vi "OAT Track Orders in Resampled Signal (Single Channel).vi"(0 "resampled signal":cluster{"r0":dbl, "dr":dbl, "Y":dbl[]}={"r0"=0.0, "dr"=1.0, "Y"=[]} {"r0" format="%.2p"; "dr" format="%.2p"; "Y" format="%.2f"}, 1 "orders (1.0)":dbl[](array[numeric])=[1.0] format="%.2f", 2 "X axis selection":u16(ring)=2 items=["Time", "Revolution", "RPM"], 3 "reset? (True)":bool=TRUE, 5 "channel info":T1={"sensor sensitivity"=1000.0, "engineering units"=1, "dB reference"=1.0, "custom label"="EU", "weighting filter"=0, "pregain"=0.0} {"pregain" format="%.2f"; "weighting filter" items=["Linear", "A-weighting", "B-weighting", "C-weighting", "ITU-R 468-4", "Dolby", "CCITT", "C-message", "Wb", "Wc", "Wd", "We", "Wf", "Wh", "Wj", "Wk", "Wm", "AES17 20 kHz lowpass", "AES17 40 kHz lowpass", "AES17 20 kHz highpass", "AES17 40 kHz highpass"]; "dB reference" format="%^.1e"; "engineering units" items=["custom..."=0, "V"=1, "A"=21, "C"=30, "pC"=31, "s"=32, "-"=29, "Pa"=2, "N"=20, "g"=3, "m/s^2"=4, "m/s"=5, "m"=6, "mm/s"=12, "mm"=13, "micron/s"=14, "micron"=15, "in/s^2"=7, "in/s"=8, "in"=9, "mil/s"=10, "mil"=11, "rad/s^2"=16, "rad/s"=17, "rad"=18, "deg/s^2"=26, "deg/s"=27, "deg"=28, "RPM"=22, "cycle/s^2"=23, "Hz"=24, "cycle"=25, "strain"=19]; "sensor sensitivity" format="%#_5f"}, 7 "time instant":dbl[](array[numeric]) format="%.2f", 11 "error in (no error)":errorcluster, 12 "bandwidth [order]":dbl format="%.2f", 13 "phase setting":T5) -> (4 "magnitudes (RMS)":cluster{"X":dbl[], "Y":dbl[]}[](array[cluster]) {"Y" format="%.2f"; "X" format="%.2f"}, 6 "phase lags":cluster{"X":dbl[], "Y":dbl[]}[](array[cluster]) {"Y" format="%.2f"; "X" format="%.2f"}, 8 "samples/rev":dbl format="%.2f", 10 "unit labels":T4, 15 "error out":errorcluster)   [LabVIEW 2017]
doc: "Computes magnitudes and phases for designated orders from <B>resampled signal</B>."
uses:
  <vilib>/addons/_NISVFA/_Shared subVIs/Controls/svc_Channel Info.ctl
  <vilib>/addons/_NISVFA/_Shared subVIs/Controls/svc_Engineering Units Text Ring.ctl
  <vilib>/addons/_NISVFA/_Shared subVIs/Controls/svc_Weighting Filter Text Ring.ctl
  <vilib>/addons/Sound and Vibration/Order Analysis/Resample Order Tracking/SubVIs/OAT Order Magnitude and Phase Plot(XY) (Single Channel).vi
  <vilib>/addons/Sound and Vibration/Order Analysis/Resample Order Tracking/SubVIs/OAT Demodulate Multiple Orders (Single Channel).vi
  <vilib>/addons/Sound and Vibration/Order Analysis/Resample Order Tracking/SubVIs/OAT Verify Resampled Signal (Single Channel).vi
  <vilib>/addons/Sound and Vibration/Order Analysis/Resample Order Tracking/SoundVib_Resampling.lvlib
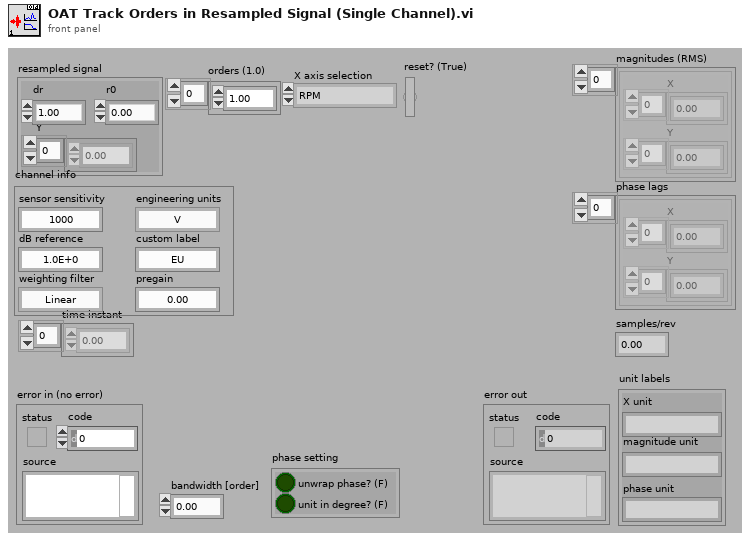
[diagram p1: front panel]
types:
  T1 = typedef "svc_Channel Info.ctl" = cluster{"sensor sensitivity":dbl, "engineering units":T2, "dB reference":dbl, "custom label":string, "weighting filter":T3, "pregain":dbl}
  T2 = typedef "svc_Engineering Units Text Ring.ctl" = u16
  T3 = typedef "svc_Weighting Filter Text Ring.ctl" = u16
  T4 = cluster{"X unit":string, "magnitude unit":string, "phase unit":string}
  T5 = cluster{"unwrap phase? (F)":bool, "unit in degree? (F)":bool}
  T6 = cluster{"bandwidth [order]":dbl, "stop band attenuation[dB]":u16}
  T7 = cluster{"X unit":string, "unit label":string, "unit label":string}
  T8 = typedef "SoundVib_TachProcess.lvlib/speed profile.ctl" = cluster{"time [s]":dbl[], "speed [RPM]":dbl[]}
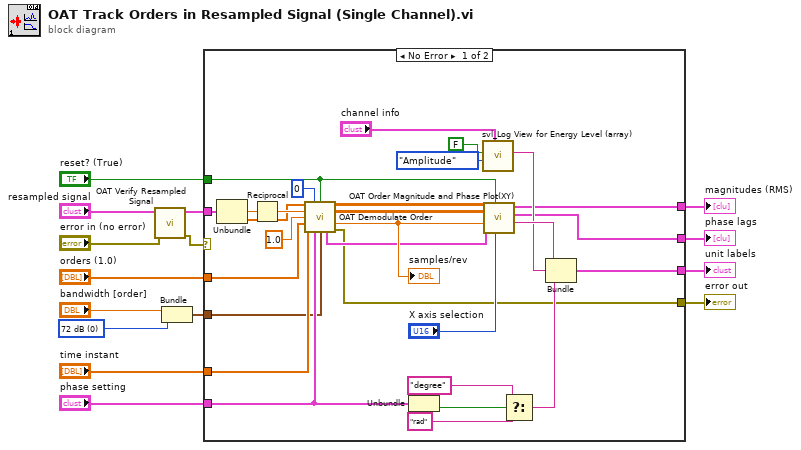
[diagram p0: block diagram]
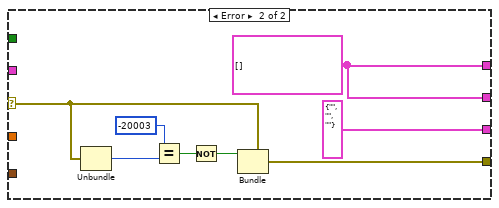
[diagram p2: hidden frame]
diagram:
  w2 = u16 0 items=["72 dB", "96 dB", "120 dB"] ("stop band attenuation[dB]")
  n1 = call-poly <vilib>:"OAT Verify Resampled Signal.vi"("error in (no error)"="error in (no error)", "resampled signal"="resampled signal") -> ("error out"=w5:errorcluster, "resampled signal dup"=w6:cluster{"r0":dbl, "dr":dbl, "Y":dbl[]})  [unwired: 7 in, 1 out]
  n2 = Bundle("bandwidth [order]"="bandwidth [order]", "stop band attenuation[dB]"=w2) -> (w1:T6)  [unwired: 1 in]
  n3 = case shown="No Error" w5 {
    selector: w5 -> [_ w46]
    tunnel: "orders (1.0)" -> [w21 _]
    tunnel: [w35 T7 {"X unit"="", "unit label"="", "unit label"=""}] -> w14
    tunnel: "time instant" -> [w34 _]
    tunnel: "phase setting" -> [w23 _]
    tunnel: [w32 w52] -> w11
    tunnel: [w28 w52] -> w10
    tunnel: "reset? (True)" -> [w26 _]
    tunnel: w6 -> [w24 _]
    tunnel: [w20 w45] -> w4
    tunnel: w1 -> [w19 _]
    frame No Error {
      n4 = Unbundle(w24) -> ("dr"=w44:dbl, "Y"=w25:dbl[])  [unwired: 1 out]
      n5 = Reciprocal(x=w44) -> (1/x=w29:dbl)
      n6 = call-poly <vilib>:"OAT Demodulate Order.vi"("Y"=w25, "decimation factor"=0 ("decimation factor (auto)"), "reset? (True)"=w26, "samples/rev"=w29, "samples/rev wanted"=1.0 ("x"), "orders (1.0)"=w21, "time stamps in"=w34, "phase setting"=w23, "order info"=w19) -> ("magnitudes (RMS)"=w27:dbl[][], "phase lag"=w31:dbl[][], "samples/rev"=w30:dbl, "speed profile"=w22:T8, "error out"=w20:errorcluster)  [unwired: 2 in]
      "samples/rev" <- w30
      n7 = Unbundle(w23) -> ("unit in degree? (F)"=w39:bool)  [unwired: 1 out]
      n8 = call <vilib>:"svl_Log View for Energy Level (array).vi"("channel info"="channel info", "view mode"=enum16{"Power", "Amplitude"}."Amplitude", "dB On (T)"=FALSE) -> ("unit label"=w40:string)  [unwired: 6 in, 2 out]
      n9 = call-poly <vilib>:"OAT Order Magnitude and Phase Plot(XY).vi"("X axis selection"="X axis selection", "reset? (True)"=w26, "speed profile"=w22, "samples/rev"=w30, "phase lag  (even angular)"=w31, "magnitudes (even angular)"=w27) -> ("X unit"=w43:string, "phase lag"=w32:cluster{"X":dbl[], "Y":dbl[]}[], "magnitudes"=w28:cluster{"X":dbl[], "Y":dbl[]}[])  [unwired: 3 in]
      n10 = Select(t="degree" ("unit label"), s=w39, f="rad" ("unit label")) -> (s? t:f=w36:string)
      n11 = Bundle("X unit"=w43, "unit label"=w40, "unit label"=w36) -> (w35:T7)  [unwired: 1 in]
    }
    frame Error {
      w52 = cluster{"X":dbl[], "Y":dbl[]}[] [] ("magnitudes")
      n12 = Unbundle(w46) -> ("code"=w50:i32)  [unwired: 2 out]
      n13 = Equal?(x=-20003 ("t"), y=w50) -> (x = y?=w48:bool)
      n14 = Not(x=w48) -> (.not. x?=w47:bool)
      n15 = Bundle(cluster=w46, "status"=w47) -> (w45:errorcluster)  [unwired: 2 in]
    }
  }
  "magnitudes (RMS)" <- w10
  "phase lags" <- w11
  "unit labels" <- w14
  "error out" <- w4
